vi "Join Strings Tree.vi"(2 "Separator (,)":string=",", 3 "Strings In":string[](array[string])) -> (0 "String":string)   [LabVIEW 2017, in "Tree API.lvlib" / "Tree.lvclass"]
doc: "Joins the elements of <B>Strings In</B> separating them with <B>Separator</B>.\n\n<B>Separator</B> - The item to put between each string.\n<B>Strings In</B> - The strings to join.\n<B>String</B> - The resultant joined string."
uses:
  Tree.lvclass
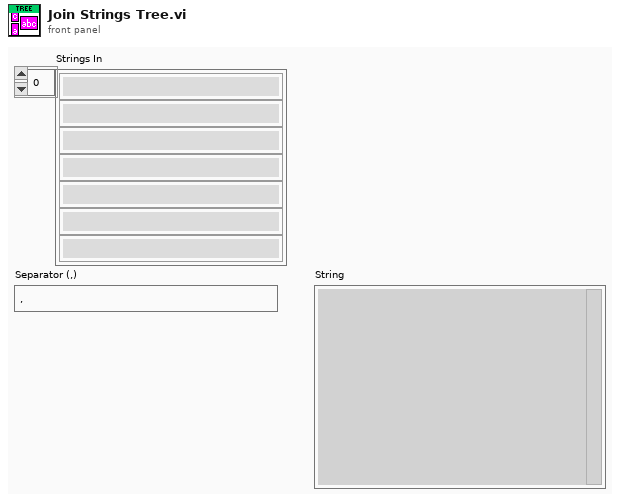
[diagram p1: front panel]
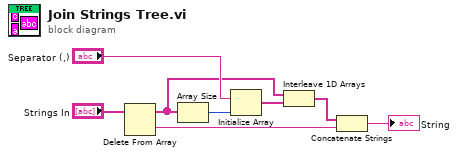
[diagram p0: block diagram]
diagram:
  n1 = Delete From Array(array="Strings In") -> (deleted portion=w2:string, array with subset deleted=w5:string[])  [unwired: 2 in]
  n2 = Array Size(array=w5) -> (size(s)=w6:i32)
  n3 = Initialize Array("Separator (,)", w6) -> (w4:string[])
  n4 = Interleave 1D Arrays(w5, w4) -> (w3:string[])
  n5 = Concatenate Strings(w3, w2) -> (→"String":string)
